vi "Generate Reference.vi"(8 "error in (no error)":errorcluster, 11 "Circular Buffer in":refnum<class "Circular Buffer.lvclass">) -> (0 "error out":errorcluster, 2 "Reference Out":refnum<data-value>, 3 "Circular Buffer Out":refnum<class "Circular Buffer.lvclass">)   [LabVIEW 2024, in "Circular Buffer.lvclass"]
uses:
  Circular Buffer.lvclass
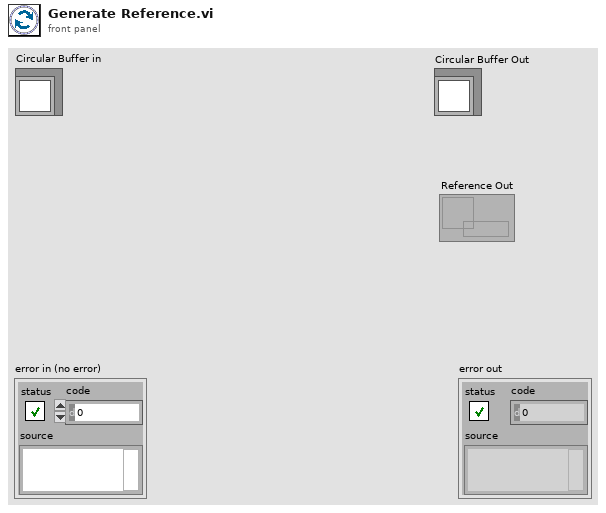
[diagram p1: front panel]
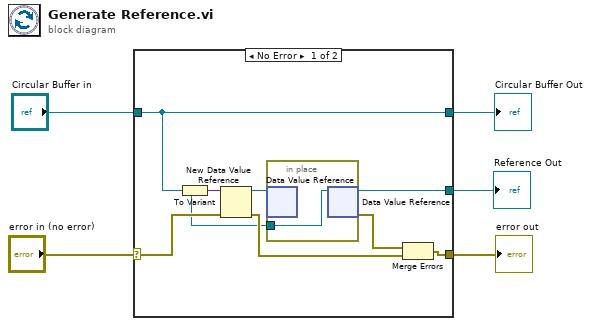
[diagram p0: block diagram]
diagram:
  n1 = case shown="No Error" "error in (no error)" {
    selector: "error in (no error)" -> [w10 w16]
    tunnel: [w7 w16] -> w4
    tunnel: "Circular Buffer in" -> [w6 w15]
    tunnel: [w11 _] -> w2
    tunnel: [w6 w15] -> w1
    frame No Error {
      n2 = To Variant(anything=w6) -> (Variant=w13:variant)
      n3 = New Data Value Reference(data value=w13, error in=w10) -> (data value reference=w12:refnum<data-value>, error out=w8:errorcluster)
      n4 = in-place {
        in-place-border: w6 -> [w14]
        n5 = in-place-dvr #1(w12) -> ()  [unwired: 2 out]
        n6 = in-place-dvr #1(w14) -> (w11:refnum<data-value>, w9:errorcluster)
      }
      n7 = Merge Errors(w9, w8) -> (w7:errorcluster)
    }
    frame Error {
    }
  }
  "error out" <- w4
  "Reference Out" <- w2
  "Circular Buffer Out" <- w1
